vi "QueueSolenAct.vi"(0 "SolenNum_IN":refnum<queue>, 5 "SolenStatue_IN":refnum<queue>, 7 "SolenNum_Value":i32, 9 "SolenStatue_Value":i32, 11 "错误输入（无错误）":errorcluster) -> (4 "SolenNum_OUT":refnum<queue>, 6 "SolenStatue_OUT":refnum<queue>, 15 "错误输出":errorcluster)   [LabVIEW 2011]
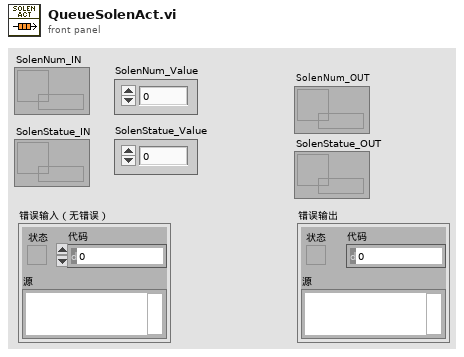
[diagram p1: front panel]
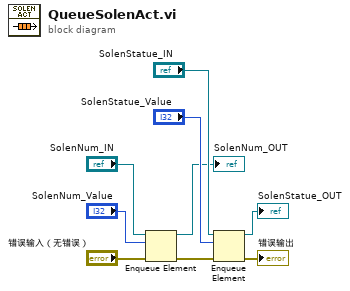
[diagram p0: block diagram]
diagram:
  n1 = Enqueue Element(queue="SolenNum_IN", element="SolenNum_Value", error in (no error)="错误输入（无错误）") -> (queue out=→"SolenNum_OUT":refnum<queue>, error out=w5:errorcluster)  [unwired: 1 in, 1 out]
  n2 = Enqueue Element(queue="SolenStatue_IN", element="SolenStatue_Value", error in (no error)=w5) -> (queue out=→"SolenStatue_OUT":refnum<queue>, error out=→"错误输出":errorcluster)  [unwired: 1 in, 1 out]
